vi "Shoot Low Goal State Machine.vi"   [LabVIEW 2013]
uses:
  typedefs/fg_typedef.ctl
  typedefs/DevRef Type.ctl
  typedefs/singleUseSubstate.ctl
  <vilib>/Rock Robotics/WPI/Solenoid/WPI_SolenoidValue.ctl
  typedefs/subStates.ctl
  <vilib>/Rock Robotics/WPI/Solenoid/WPI_SolenoidGetEnum.vi
panel:
  # "A State Machine to Handle a Low Goal Shot"
types:
  T1 = typedef "DevRef Type.ctl" = enum16{"Shooter Solenoid", "Latch Solenoid", "Right Up Sensor", "Right Down Sensor", "Hold Sensor", "Arm Encoder"}
  T2 = typedef "fg_typedef.ctl" = enum16{"Get", "Set"}
  T3 = typedef "WPI_SolenoidValue.ctl" = enum16{"Off", "On", "Forward", "Reverse"}
  T4 = typedef "singleUseSubstate.ctl" = enum16{"null", "wait", "shift high", "shift low", "extend shooter", "retract shooter", "latch", "unlatch"}
  T5 = typedef "subStates.ctl" = enum16{"null", "wait", "driver control", "auto", "manual override", "hold position", "rotate", "pickup", "pass", "load", "goto shoot", "shoot high goal", "shoot low goal", "cancel arm", "cancel shooter", "end"}
  T6 = typedef "WPI_DigitalInputDevRef.ctl" = cluster{"DevStatus":errorcluster, "DIO Channel":T7, "Digital Module":T8}
  T7 = typedef "FPGA_DIOChannel.ctl" = enum8{"DIO 1", "DIO 2", "DIO 3", "DIO 4", "DIO 5", "DIO 6", "DIO 7", "DIO 8", "DIO 9", "DIO 10", "DIO 11", "DIO 12", "DIO 13", "DIO 14", "Invalid"}
  T8 = typedef "FPGA_TypedefDigitalModule.ctl" = enum16{"Digital Module 1", "Digital Module 2"}
  T9 = typedef "WPI_SolenoidDevRef.ctl" = cluster{"DevStatus":errorcluster, "Solenoid Module":T10, "Forward Solenoid Channel":T11, "Reverse Solenoid Channel":T11}
  T10 = typedef "FPGA_TypedefSolenoidModule.ctl" = enum16{"Solenoid Module 1", "Solenoid Module 2"}
  T11 = typedef "WPI_SolenoidChannel.ctl" = enum8{"Solenoid 1", "Solenoid 2", "Solenoid 3", "Solenoid 4", "Solenoid 5", "Solenoid 6", "Solenoid 7", "Solenoid 8", "Invalid"}
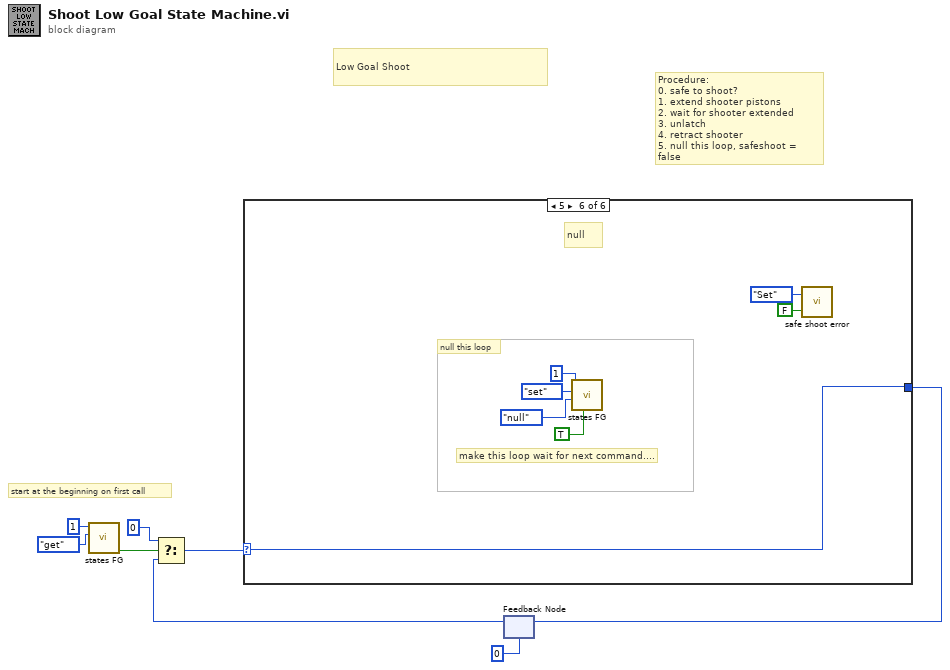
[diagram p0: block diagram]
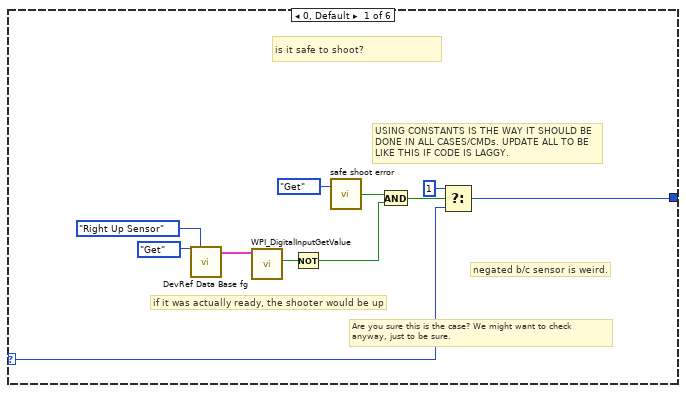
[diagram p2: hidden frame]
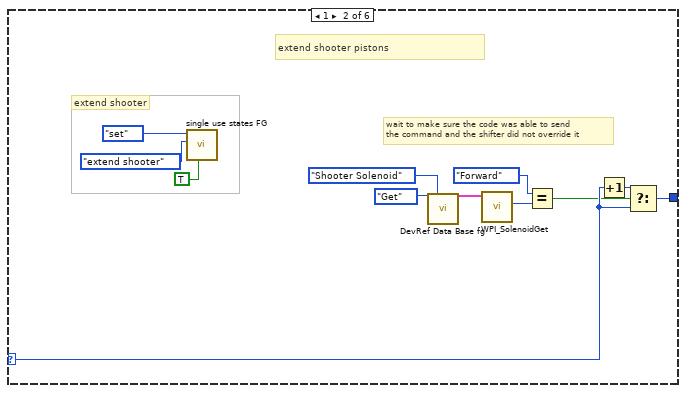
[diagram p3: hidden frame]
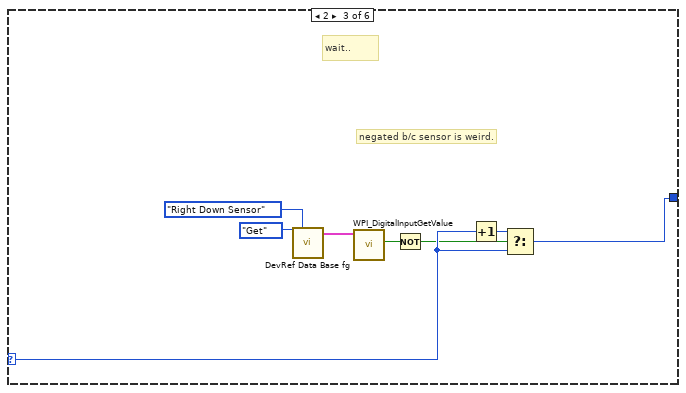
[diagram p4: hidden frame]
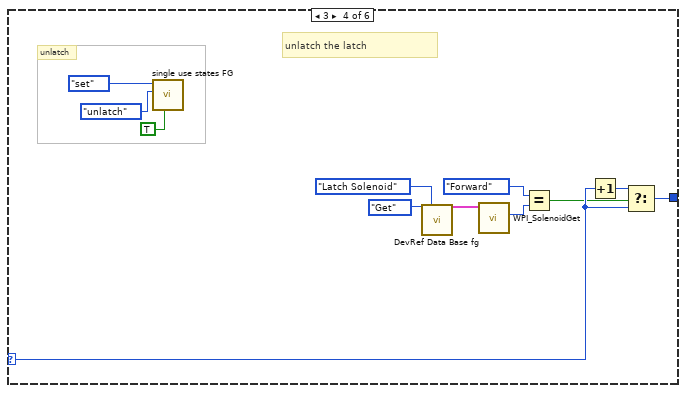
[diagram p5: hidden frame]
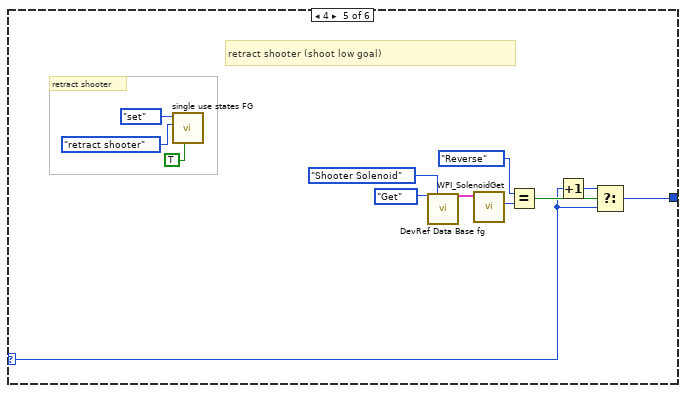
[diagram p6: hidden frame]
diagram:
  # "start at the beginning on first call"
  # "Low Goal Shoot"
  # "Procedure:\n0. safe to shoot? \n1. extend shooter pistons\n2. wait for shooter extended\n3. unlatch\n4. retract shooter\n5. null this loop, safeshoot = false"
  n1 = call "states FG.vi"("menu (get)"=enum16{"set", "get"}."get", "Loop ID"=1) -> ("first call?"=w1:bool)  [unwired: 6 in, 3 out]
  n2 = feedback #1(u8 0) -> (w4:u8)
  n3 = Select(t=u8 0, s=w1, f=w4) -> (s? t:f=w3:u8)
  n4 = case shown="5" w3 {
    selector: w3 -> [w9 w27 w37 w46 w53 w70]
    tunnel: [w17 w25 w36 w47 w55 w70] -> w7
    frame 0, Default {
      # "negated b/c sensor is weird."
      # "Are you sure this is the case? We might want to check\nanyway, just to be sure."
      # "USING CONSTANTS IS THE WAY IT SHOULD BE\nDONE IN ALL CASES/CMDs. UPDATE ALL TO BE\nLIKE THIS IF CODE IS LAGGY."
      # "if it was actually ready, the shooter would be up"
      # "is it safe to shoot?"
      n5 = call "DevRef Data Base fg.vi"("Menu"=fg_typedef."Get", "DevRef to Get"=DevRef_Type."Right Up Sensor") -> ("Selected Sensor"=w13:T6)  [unwired: 23 in, 2 out]
      n6 = call <vilib>:"WPI_DigitalInputGetValue.vi"("DigitalInputDevRef"=w13) -> ("Value"=w15:bool)  [unwired: 8 in, 2 out]
      n7 = Not(x=w15) -> (.not. x?=w10:bool)
      n8 = call "safe shoot error.vi"("Menu"=fg_typedef."Get") -> ("Can Shoot Safely?"=w18:bool)  [unwired: 1 in]
      n9 = And(x=w18, y=w10) -> (x .and. y?=w11:bool)
      n10 = Select(t=u8 1, s=w11, f=w9) -> (s? t:f=w17:u8)
    }
    frame 1 {
      # "wait to make sure the code was able to send\nthe command and the shifter did not override it"
      # "extend shooter"
      # "extend shooter pistons"
      n11 = call "single use states FG.vi"("exit in"=TRUE, "substate"=singleUseSubstate."extend shooter", "menu (get)"=enum16{"set", "get"}."set") -> ()  [unwired: 5 in, 4 out]
      n12 = call "DevRef Data Base fg.vi"("Menu"=fg_typedef."Get", "DevRef to Get"=DevRef_Type."Shooter Solenoid") -> ("Selected Solenoid"=w24:T9)  [unwired: 23 in, 2 out]
      n13 = call-poly <vilib>:"WPI_SolenoidGet.vi"("SolenoidDevRef"=w24) -> ("Value"=w23:T3)  [unwired: 8 in, 2 out]
      n14 = Equal?(x=WPI_SolenoidValue."Forward" ("Value"), y=w23) -> (x = y?=w21:bool)
      n15 = Increment(x=w27) -> (x+1=w26:u8)
      n16 = Select(t=w26, s=w21, f=w27) -> (s? t:f=w25:u8)
    }
    frame 2 {
      # "negated b/c sensor is weird."
      # "wait.."
      n17 = call "DevRef Data Base fg.vi"("Menu"=fg_typedef."Get", "DevRef to Get"=DevRef_Type."Right Down Sensor") -> ("Selected Sensor"=w34:T6)  [unwired: 23 in, 2 out]
      n18 = call <vilib>:"WPI_DigitalInputGetValue.vi"("DigitalInputDevRef"=w34) -> ("Value"=w38:bool)  [unwired: 8 in, 2 out]
      n19 = Not(x=w38) -> (.not. x?=w32:bool)
      n20 = Increment(x=w37) -> (x+1=w39:u8)
      n21 = Select(t=w39, s=w32, f=w37) -> (s? t:f=w36:u8)
    }
    frame 3 {
      # "unlatch the latch"
      # "unlatch"
      n22 = call "single use states FG.vi"("exit in"=TRUE, "substate"=singleUseSubstate."unlatch", "menu (get)"=enum16{"set", "get"}."set") -> ()  [unwired: 5 in, 4 out]
      n23 = call "DevRef Data Base fg.vi"("Menu"=fg_typedef."Get", "DevRef to Get"=DevRef_Type."Latch Solenoid") -> ("Selected Solenoid"=w44:T9)  [unwired: 23 in, 2 out]
      n24 = call-poly <vilib>:"WPI_SolenoidGet.vi"("SolenoidDevRef"=w44) -> ("Value"=w43:T3)  [unwired: 8 in, 2 out]
      n25 = Equal?(x=WPI_SolenoidValue."Forward" ("Value"), y=w43) -> (x = y?=w41:bool)
      n26 = Increment(x=w46) -> (x+1=w45:u8)
      n27 = Select(t=w45, s=w41, f=w46) -> (s? t:f=w47:u8)
    }
    frame 4 {
      # "retract shooter"
      # "retract shooter (shoot low goal)"
      n28 = call "single use states FG.vi"("exit in"=TRUE, "substate"=singleUseSubstate."retract shooter", "menu (get)"=enum16{"set", "get"}."set") -> ()  [unwired: 5 in, 4 out]
      n29 = call "DevRef Data Base fg.vi"("Menu"=fg_typedef."Get", "DevRef to Get"=DevRef_Type."Shooter Solenoid") -> ("Selected Solenoid"=w59:T9)  [unwired: 23 in, 2 out]
      n30 = call-poly <vilib>:"WPI_SolenoidGet.vi"("SolenoidDevRef"=w59) -> ("Value"=w58:T3)  [unwired: 8 in, 2 out]
      n31 = Equal?(x=WPI_SolenoidValue."Reverse" ("Value"), y=w58) -> (x = y?=w56:bool)
      n32 = Increment(x=w53) -> (x+1=w54:u8)
      n33 = Select(t=w54, s=w56, f=w53) -> (s? t:f=w55:u8)
    }
    frame 5 {
      # "null this loop"
      # "make this loop wait for next command...."
      # "null"
      n34 = call "states FG.vi"("exit in"=TRUE, "subState in"=subStates."null", "menu (get)"=enum16{"set", "get"}."set", "Loop ID"=1) -> ()  [unwired: 4 in, 4 out]
      n35 = call "safe shoot error.vi"("Can Shoot Safely?"=FALSE, "Menu"=fg_typedef."Set") -> ()  [unwired: 1 out]
    }
  }
  n36 = feedback-in #1(w7) -> ()
